vi "Create Low Pass Filter (FGV).vi"(6 "fs (Hz)":dbl, 7 "init [F]":bool, 8 "error in (no error)":errorcluster, 9 "Low Pass Cutoff (Hz)":dbl, 11 "order":i32=2) -> (0 "error out":errorcluster, 3 "IIR Filters":T1(array[cluster]), 5 "init out":bool)   [LabVIEW 2019, in "DSP.lvclass"]
uses:
  DSP.lvclass
  <vilib>/Analysis/3filter.llb/Filter Passband Type.ctl
  <vilib>/Analysis/NI_AALBase.lvlib
panel:
  out "concatenated string":string
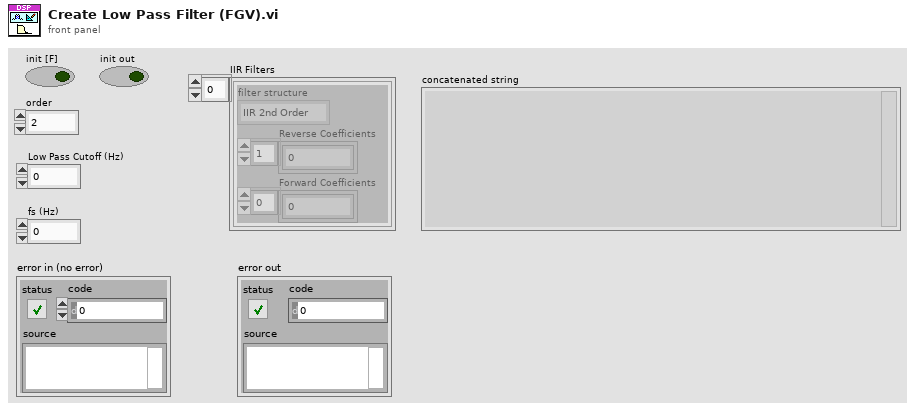
[diagram p1: front panel]
types:
  T1 = cluster{"filter structure":enum32{"IIR 2nd Order", "IIR 4th Order"}, "Reverse Coefficients":dbl[], "Forward Coefficients":dbl[]}[]
  T2 = typedef "NI_AALBase.lvlib/Filter Passband Type.ctl" = enum32{"Lowpass", "Highpass", "Bandpass", "Bandstop"}
  T3 = cluster{"filter structure":enum32{"IIR 2nd Order", "IIR 4th Order"}, "Reverse Coefficients":dbl[], "Forward Coefficients":dbl[]}
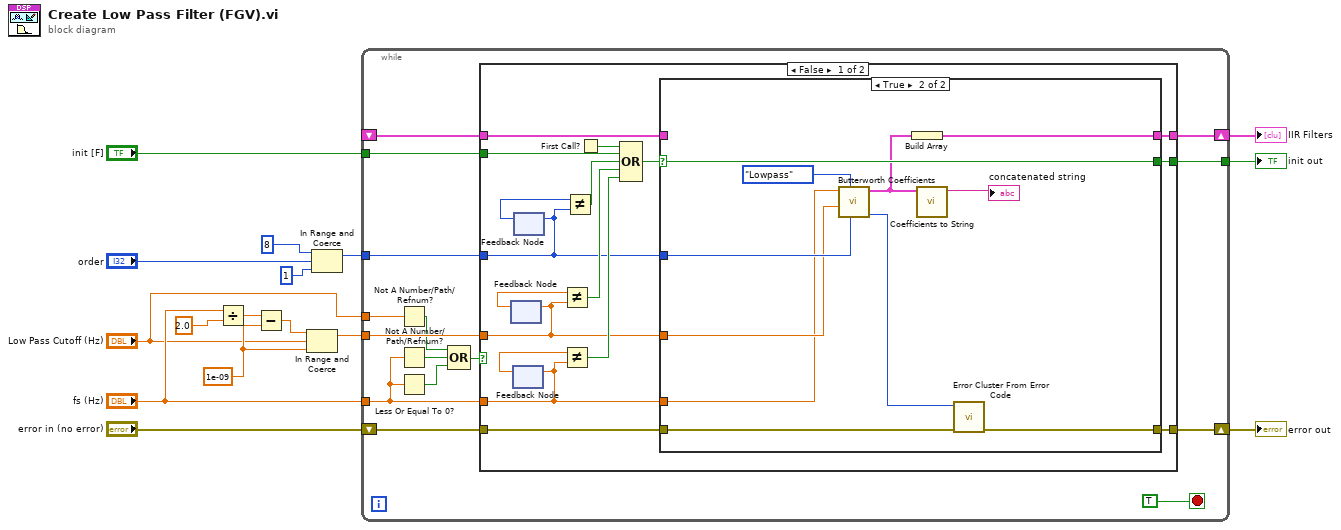
[diagram p0: block diagram]
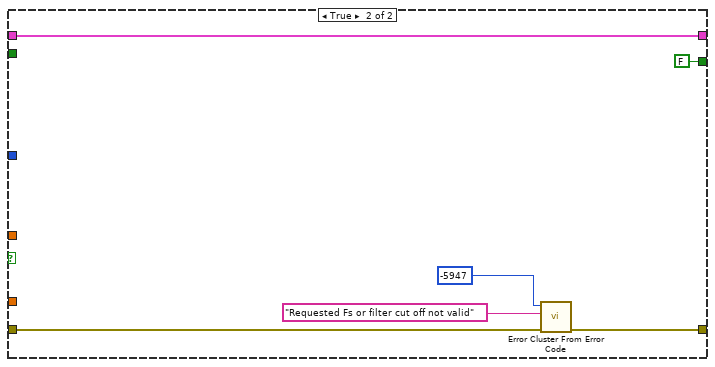
[diagram p3: hidden frame]
diagram:
  w3 = 1e-09 ("lower limit")
  n1 = Divide(x="fs (Hz)", y=2.0 ("lower limit")) -> (x/y=w14:dbl)
  n2 = Subtract(x=w14, y=w3) -> (x-y=w13:dbl)
  n3 = In Range and Coerce(upper limit=w13, x="Low Pass Cutoff (Hz)", lower limit=w3) -> (coerced(x)=w10:dbl)  [unwired: 1 out]
  n4 = In Range and Coerce(upper limit=8, x="order", lower limit=1) -> (coerced(x)=w6:i32)  [unwired: 1 out]
  n5 = while {
    tunnel: w10 -> [w22]
    tunnel: "fs (Hz)" -> [w23]
    shift-right: [w29] -> w16
    shift-left: "error in (no error)" -> [w30]
    shift-right: [w31] -> w2
    shift-left: _ -> [w27]
    tunnel: "init [F]" -> [w26]
    tunnel: w6 -> [w25]
    tunnel: [w24] -> w4
    tunnel: "Low Pass Cutoff (Hz)" -> [w17]
    stop <- TRUE stop-if-true
    n6 = Not A Number/Path/Refnum?(number/path/refnum=w17) -> (NaN/Path/Refnum?=w21:bool)
    n7 = Not A Number/Path/Refnum?(number/path/refnum=w23) -> (NaN/Path/Refnum?=w20:bool)
    n8 = Less Or Equal To 0?(x=w23) -> (x <= 0?=w19:bool)
    n9 = Compound Arithmetic op=OR(w21, w20, w19) -> (w18:bool)
    n10 = case shown="False" w18 {
      tunnel: [w48 w68] -> w31
      tunnel: w30 -> [w47 w65]
      tunnel: [w46 w66] -> w29
      tunnel: w27 -> [w44 w68]
      tunnel: w26 -> [w43 _]
      tunnel: w25 -> [w36 _]
      tunnel: [w34 FALSE] -> w24
      tunnel: w23 -> [w33 _]
      tunnel: w22 -> [w32 _]
      frame False {
        n11 = feedback #1() -> (w40:dbl)  [unwired: 1 in]
        n12 = feedback-in #1(w32) -> ()
        n13 = feedback #2() -> (w41:dbl)  [unwired: 1 in]
        n14 = feedback-in #2(w33) -> ()
        n15 = feedback #3() -> (w39:i32)  [unwired: 1 in]
        n16 = feedback-in #3(w36) -> ()
        n17 = Not Equal?(x=w40, y=w32) -> (x != y?=w45:bool)
        n18 = Not Equal?(x=w41, y=w33) -> (x != y?=w38:bool)
        n19 = Not Equal?(x=w39, y=w36) -> (x != y?=w37:bool)
        n20 = First Call?() -> (First Call?: T/F=w35:bool)
        n21 = Compound Arithmetic op=OR(w35, w43, w37, w45, w38) -> (w42:bool)
        n22 = case shown="True" w42 {
          selector: w42 -> [w49 w62]
          tunnel: [w51 w57] -> w48
          tunnel: w47 -> [w50 w59]
          tunnel: [w50 w60] -> w46
          tunnel: w32 -> [_ w55]
          tunnel: w33 -> [_ w53]
          tunnel: w44 -> [w51 _]
          tunnel: w36 -> [_ w56]
          tunnel: [w49 w62] -> w34
          frame False {
          }
          frame True {
            n23 = call <vilib>:"Butterworth Coefficients.vi"("order"=w56, "filter type"=Filter_Passband_Type."Lowpass", "low cutoff freq: fl"=w55, "sampling freq: fs"=w53) -> ("error"=w58:i32, "IIR Filter Cluster"=w52:T3)  [unwired: 6 in]
            n24 = Build Array(w52) -> (w57:T1)
            n25 = call "Coefficients to String.vi"("IIR Filter Cluster"=w52) -> ("String"=→"concatenated string":string)  [unwired: 10 in]
            n26 = call <vilib>:"Error Cluster From Error Code.vi"("error in (no error)"=w59, "error code (0)"=w58) -> ("error out"=w60:errorcluster)  [unwired: 7 in]
          }
        }
      }
      frame True {
        n27 = call <vilib>:"Error Cluster From Error Code.vi"("error in (no error)"=w65, "error message (\"\")"="Requested Fs or filter cut off not valid" ("error message (\"\")"), "error code (0)"=-5947) -> ("error out"=w66:errorcluster)  [unwired: 6 in]
      }
    }
  }
  "init out" <- w4
  "IIR Filters" <- w2
  "error out" <- w16
